vi "Temperaturas.vi"() -> ()   [LabVIEW 2017]
panel:
  in  "Temperaturas":T1
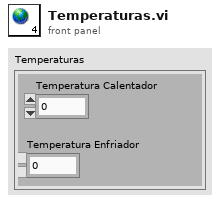
[diagram p1: front panel]
types:
  T1 = cluster{"Temperatura Calentador":dbl, "Temperatura Enfriador":dbl}
diagram:
